vi "Configure IF Bandwith.vi"(8 "error in (no error)":errorcluster, 10 "IF BW [Hz]":dbl, 11 "Vector Network Analyzer in":refnum<class "Vector Network Analyzer.lvclass">) -> (0 "error out":errorcluster, 2 "IF BW used [Hz]":dbl, 3 "Vector Network Analyzer out":refnum<class "Vector Network Analyzer.lvclass">)   [LabVIEW 2020, in "Vector Network Analyzer.lvclass"]
doc: "Configures the Intermidiate Frequency Bandwidth. \nIt chooses the closest supported bandwidth.\nIt returns the used IF BW."
uses:
  Vector Network Analyzer.lvclass
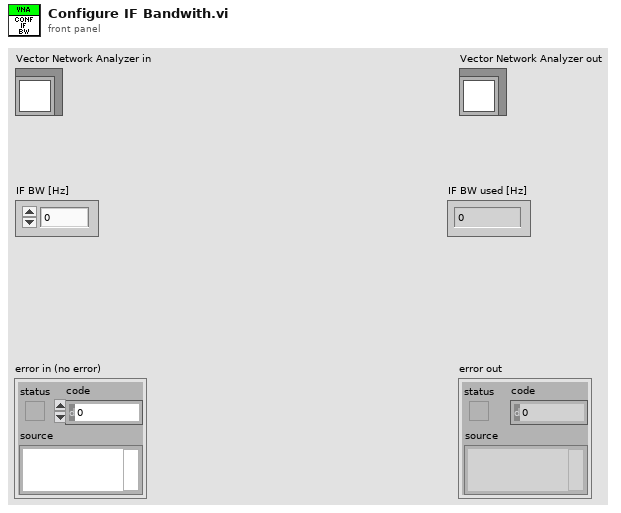
[diagram p1: front panel]
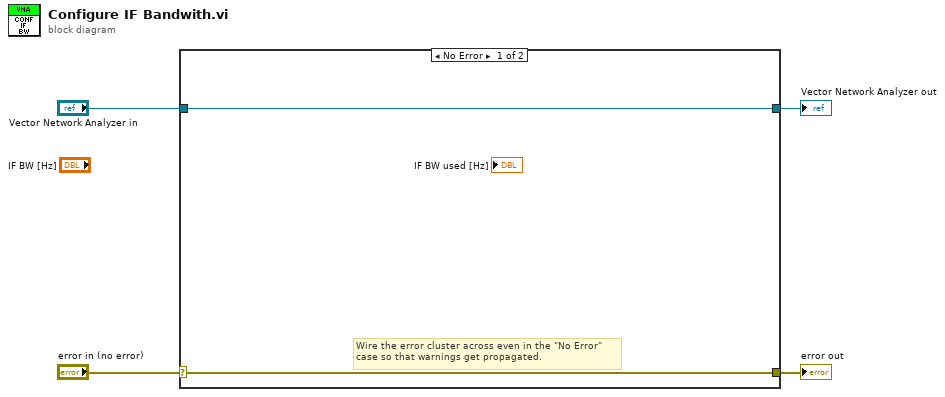
[diagram p0: block diagram]
diagram:
  n1 = case shown="No Error" "error in (no error)" {
    selector: "error in (no error)" -> [w5 w8]
    tunnel: [w5 w8] -> w3
    tunnel: [w6 w7] -> w1
    tunnel: "Vector Network Analyzer in" -> [w6 w7]
    frame No Error {
      # "Wire the error cluster across even in the \"No Error\"\ncase so that warnings get propagated."
    }
    frame Error {
    }
  }
  "error out" <- w3
  "Vector Network Analyzer out" <- w1
